vi "Draw Steering Wheel.vi"(6 "wheel state":T1, 7 "picture info":T3={"picture size"={"Width"=500, "Height"=500}, "pixels per unit"=10.0}, 8 "error in (no error)":errorcluster, 9 "draw wheel options":T2={"global wheel position"={"x"=0.0, "y"=0.0}, "wheel frame angle (rad)"=0.0, "color (black)"=0, "draw wheel state"=FALSE, "draw forward velocity"=FALSE, "velocity scale"=16711680.0, "velocity color (red)"=16711680}, 10 "picture in":picture, 11 "wheel in":refnum<class "NI_Robotics_Wheel.lvclass">) -> (0 "error out":errorcluster, 2 "picture out":picture, 3 "wheel out":refnum<class "NI_Robotics_Wheel.lvclass">)   [LabVIEW 2017, in "NI_Robotics_Steering Picture.lvlib"]
uses:
  <vilib>/robotics/Utilities/Visualization/Steering Visualization/Steering Picture/NI_Robotics_Steering Picture.lvlib
  <vilib>/robotics/Steering/Wheel/NI_Robotics_Wheel.lvclass
  <vilib>/robotics/Utilities/Visualization/Steering Visualization/Steering Picture/Picture Info.ctl
  <vilib>/Utility/miscctls.llb/LVBoundsTypeDef.ctl
  <vilib>/robotics/Utilities/Visualization/Steering Visualization/Steering Picture/Draw Wheel Options.ctl
  <vilib>/robotics/Steering/Wheel/Wheel State.ctl
  <vilib>/Analysis/coordinate.llb/Angle Rotation (scalar).vi
  <vilib>/Analysis/coordinate.llb/2D Cartesian Coordinate Rotation.vi
  <vilib>/Analysis/coordinate.llb/2D Cartesian Coordinate Rotation (Array).vi
  <vilib>/robotics/Utilities/Visualization/Steering Visualization/Steering Picture/Global Position to Pixel.vi
  <vilib>/Analysis/coordinate.llb/Wrap Angle.vi
  <vilib>/Analysis/coordinate.llb/Wrap Angle (scalar).vi
  <vilib>/picture/picture.llb/Draw Line.vi
  <vilib>/picture/picture.llb/Move Pen.vi
  <vilib>/picture/picture.llb/Draw Point.vi
  <vilib>/picture/picture.llb/Draw Multiple Lines.vi
  <vilib>/picture/pictutil.llb/Draw Circle by Radius.vi
  <vilib>/Utility/AngleManip/Radians to Degrees.vi
  <vilib>/Utility/AngleManip/Radians to Degrees (Scalar DBL).vi
  <vilib>/robotics/Steering/Wheel/Get Steering Wheel Information.vi
  <vilib>/Analysis/NI_AAL_Angle.lvlib
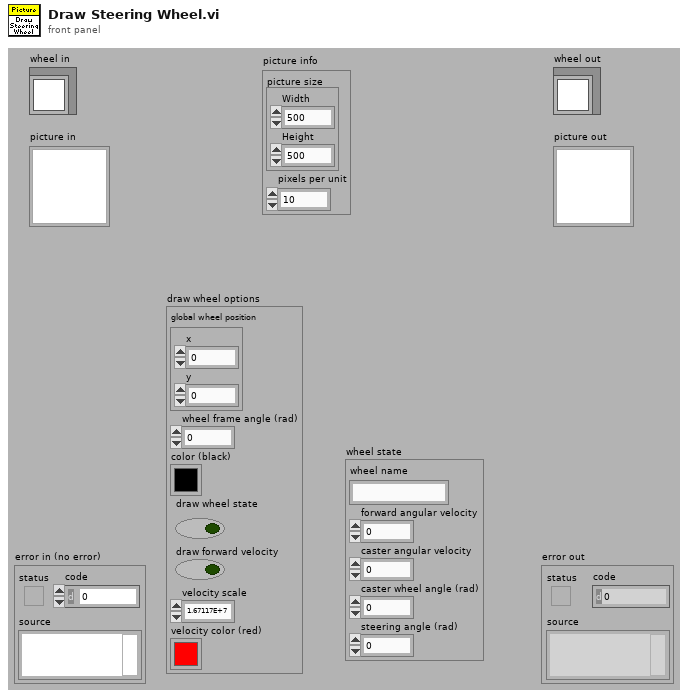
[diagram p1: front panel]
types:
  T1 = typedef "NI_Robotics_Wheel.lvclass/Wheel State.ctl" = cluster{"wheel name":string, "forward angular velocity":dbl, "caster angular velocity":dbl, "caster wheel angle (rad)":dbl, "steering angle (rad)":dbl}
  T2 = typedef "NI_Robotics_Steering Picture.lvlib/Draw Wheel Options.ctl" = cluster{"global wheel position":cluster{"x":dbl, "y":dbl}, "wheel frame angle (rad)":dbl, "color (black)":u32, "draw wheel state":bool, "draw forward velocity":bool, "velocity scale":dbl, "velocity color (red)":u32}
  T3 = typedef "NI_Robotics_Steering Picture.lvlib/Picture Info.ctl" = cluster{"picture size":T4, "pixels per unit":dbl}
  T4 = typedef "LVBoundsTypeDef.ctl" = cluster{"Width":u32, "Height":u32}
  T5 = typedef "NI_Robotics_Wheel.lvclass/Wheel Parameters.ctl" = cluster{"wheel radius":dbl, "gear ratio":dbl, "forward rotation direction":T6}
  T6 = typedef "NI_Robotics_Wheel.lvclass/Rotation Direction.ctl" = u16
  T7 = typedef "NI_Robotics_Steering Wheel.lvclass/Steering Wheel Parameters.ctl" = cluster{"steering gear ratio":dbl, "motor angle offset (rad)":dbl, "steering angle range":T8}
  T8 = typedef "NI_Robotics_Steering Wheel.lvclass/Steering Angle Range.ctl" = cluster{"min steering angle (rad)":dbl, "max steering angle (rad)":dbl}
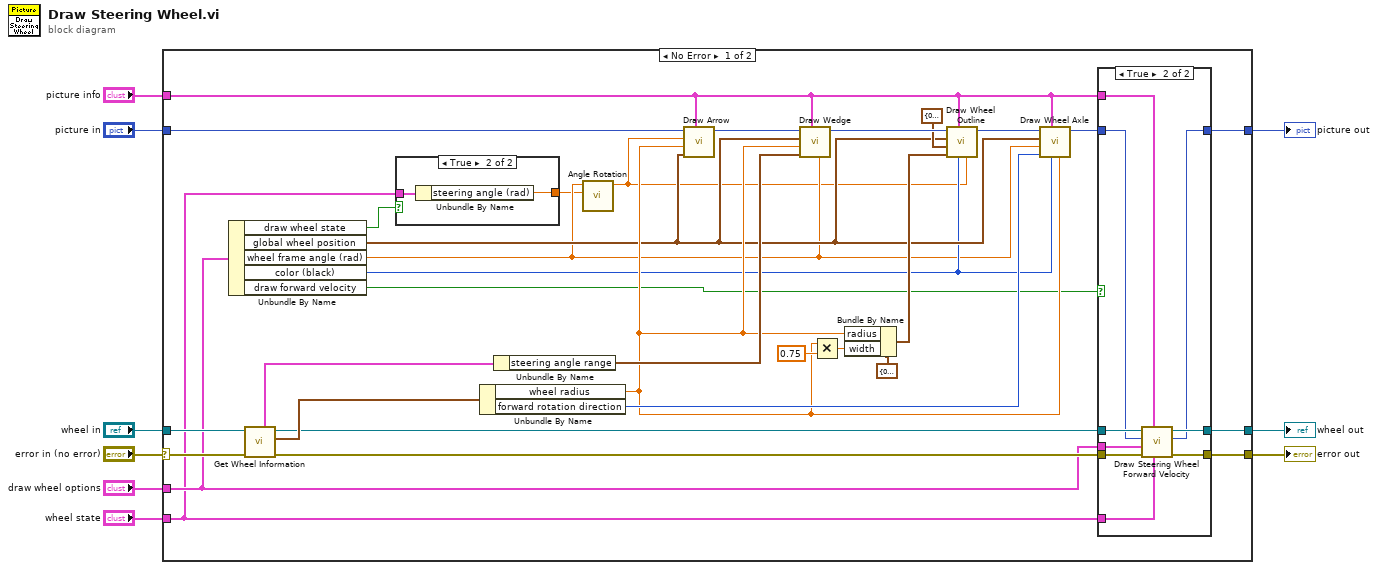
[diagram p0: block diagram]
diagram:
  n1 = case shown="No Error" "error in (no error)" {
    selector: "error in (no error)" -> [w40 w58]
    tunnel: [w20 w58] -> w5
    tunnel: "wheel in" -> [w41 w56]
    tunnel: "picture in" -> [w39 w57]
    tunnel: [w18 w57] -> w7
    tunnel: [w22 w56] -> w6
    tunnel: "picture info" -> [w17 _]
    tunnel: "draw wheel options" -> [w15 _]
    tunnel: "wheel state" -> [w14 _]
    frame No Error {
      n2 = Unbundle By Name(w15) -> ("draw wheel state"=w13:bool, "global wheel position"=w25:cluster{"x":dbl, "y":dbl}, "wheel frame angle (rad)"=w12:dbl, "color (black)"=w24:u32, "draw forward velocity"=w16:bool)
      n3 = call-poly <vilib>:"Get Wheel Information.vi"("error in (no error)"=w40, "wheel in"=w41) -> ("error out"=w21:errorcluster, "wheel parameters"=w37:T5, "wheel out"=w23:refnum<class "NI_Robotics_Wheel.lvclass">, "steering parameters"=w36:T7)  [unwired: 3 in, 3 out]
      n4 = case shown="True" w13 {
        tunnel: [_ w43] -> w10
        tunnel: w14 -> [_ w42]
        frame False {
        }
        frame True {
          n5 = Unbundle By Name(w42) -> ("steering angle (rad)"=w43:dbl)
        }
      }
      n6 = Unbundle By Name(w37) -> ("wheel radius"=w27:dbl, "forward rotation direction"=w28:T6)
      n7 = Unbundle By Name(w36) -> ("steering angle range"=w35:T8)
      n8 = call-poly <vilib>:"Angle Rotation.vi"("counterclockwise rotation"=w10, "angle"=w12) -> ("rotated angle"=w11:dbl)  [unwired: 8 in, 1 out]
      n9 = call <vilib>:"Draw Arrow.vi"("picture info"=w17, "global base position"=w25, "length"=w27, "wheel frame angle (rad)"=w11, "picture in"=w39) -> ("picture out"=w38:picture)  [unwired: 6 in]
      n10 = call <vilib>:"Draw Wedge.vi"("wheel frame angle (rad)"=w12, "picture info"=w17, "steering angle range"=w35, "radius"=w27, "global wheel position"=w25, "picture in"=w38) -> ("picture out"=w34:picture)  [unwired: 5 in]
      n11 = Multiply(x=w27, y=0.75) -> (x*y=w33:dbl)
      n12 = Bundle By Name(cluster=cluster{"radius":dbl, "width":dbl} {"radius"=0.0, "width"=0.0} ("size"), "radius"=w27, "width"=w33) -> (w30:cluster{"radius":dbl, "width":dbl})
      n13 = call <vilib>:"Draw Wheel Outline.vi"("angle (rad)"=w11, "color (black)"=w24, "picture info"=w17, "size"=w30, "offset from center"=cluster{"x":dbl, "y":dbl} {"x"=0.0, "y"=0.0}, "global wheel position"=w25, "picture in"=w34) -> ("picture out"=w29:picture)  [unwired: 4 in]
      n14 = call <vilib>:"Draw Wheel Axle.vi"("length"=w27, "color (black)"=w24, "picture info"=w17, "rotation direction"=w28, "wheel frame angle (rad)"=w12, "global wheel position"=w25, "picture in"=w29) -> ("picture out"=w19:picture)  [unwired: 4 in]
      n15 = case shown="True" w16 {
        tunnel: w23 -> [w45 w55]
        tunnel: [w45 w54] -> w22
        tunnel: w21 -> [w44 w53]
        tunnel: [w44 w52] -> w20
        tunnel: w19 -> [w46 w51]
        tunnel: [w46 w50] -> w18
        tunnel: w17 -> [_ w49]
        tunnel: w15 -> [_ w48]
        tunnel: w14 -> [_ w47]
        frame False {
        }
        frame True {
          n16 = call <vilib>:"Draw Steering Wheel Forward Velocity.vi"("wheel state"=w47, "picture info"=w49, "error in (no error)"=w53, "draw wheel options"=w48, "picture in"=w51, "wheel in"=w55) -> ("error out"=w52:errorcluster, "picture out"=w50:picture, "wheel out"=w54:refnum<class "NI_Robotics_Wheel.lvclass">)  [unwired: 3 in]
        }
      }
    }
    frame Error {
    }
  }
  "error out" <- w5
  "wheel out" <- w6
  "picture out" <- w7
